vi "gxml_RcrsvParse.vi"(6 "File Item Contents":string, 7 "Empty XML Array?":bool, 8 "error in":errorcluster, 9 "Flat String In":string, 11 "Item TypeDesc":variant) -> (0 "error out":errorcluster, 1 "Flat String Out":string)   [LabVIEW 2011, in "Third Party VIs.lvlib" / "GXML.lvlib"]
doc: "This recursive VI is the core engine responsible for searching the XML string. The VI recursively dives into the type definition cluster and identifies individual elements by name. In parallel the VI also looks at the XML string for tags that have the same name and hierarchy. If a match is found the data is extracted from the XML file and appropriately inserted into a flattened data string."
uses:
  GXML.lvlib
  <vilib>/Utility/VariantDataType/VariantType.lvlib
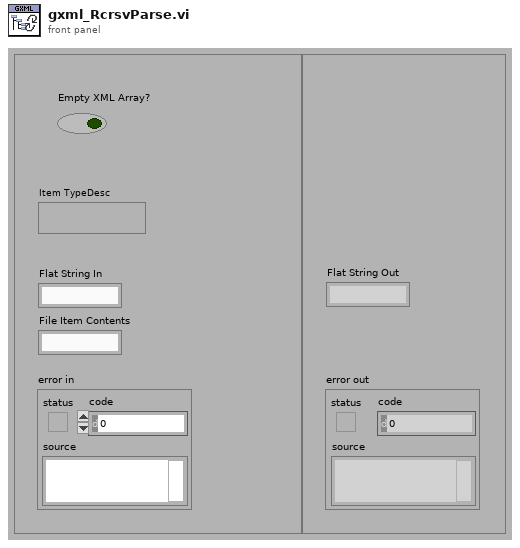
[diagram p1: front panel]
types:
  T1 = typedef "VariantType.lvlib/Type.ctl" = enum8{"Invalid Type", "Void", "I8", "I16", "I32", "I64", "U8", "U16", "U32", "U64", "Single Float", "Double Float", "Extended Float", "Single Complex", "Double Complex", "Extended Complex", "Enum U8", "Enum U16", "Enum U32", "Enum U64", "Single Float With Unit", "Double Float With Unit", "Extended Float With Unit", "Single Complex with Unit", "Double Complex with Unit", "Extended Complex with Unit", "Boolean", "String", "Path", "Picture", "Tag", "Array", "Cluster", "Variant", "LV Variant", "Waveform", "Timestamp", "Digital Waveform", "Digital Data", "ExpressData", "Refnum", "External Data", "VI", "Poly VI", "LabVIEW Class Instance", "Fixed Point"}
  T2 = cluster{"Item 'Name'":string, "Item Attributes":string, "Item Contents":string}
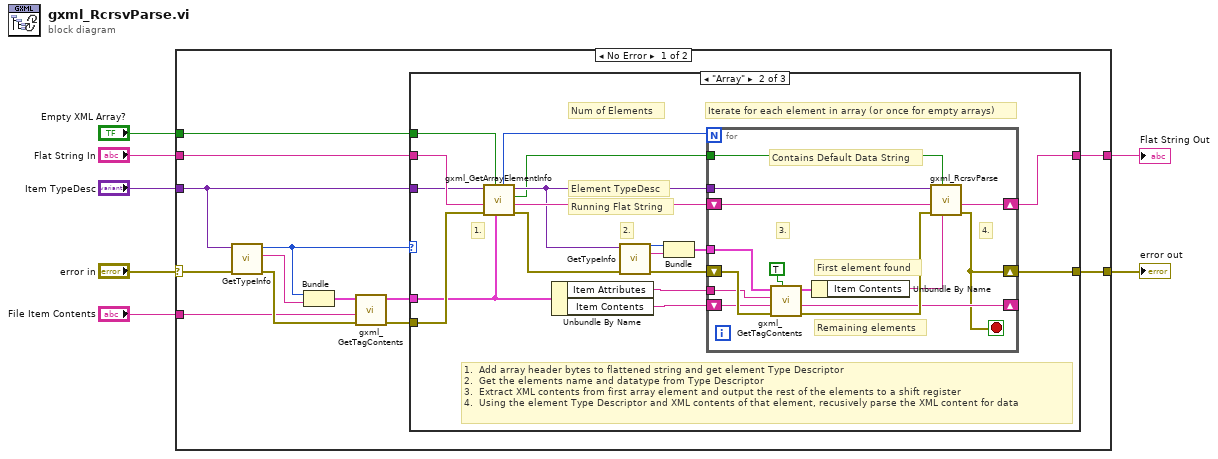
[diagram p0: block diagram]
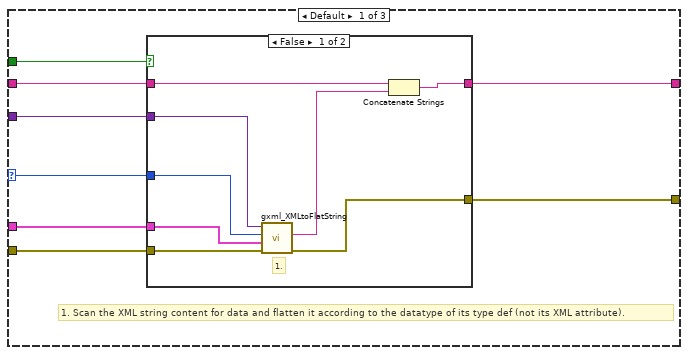
[diagram p2: hidden frame]
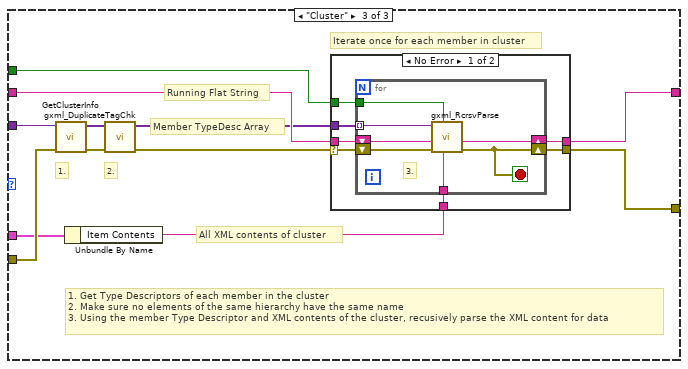
[diagram p4: hidden frame]
diagram:
  n1 = case shown="No Error" "error in" {
    selector: "error in" -> [w19 w100]
    tunnel: [w20 w100] -> w7
    tunnel: "File Item Contents" -> [w13 _]
    tunnel: "Item TypeDesc" -> [w18 _]
    tunnel: "Flat String In" -> [w9 w99]
    tunnel: [w17 w99] -> w3
    tunnel: "Empty XML Array?" -> [w8 _]
    frame No Error {
      n2 = call <vilib>:"GetTypeInfo.vi"("error in (no error)"=w19, "Variant"=w18) -> ("error out"=w16:errorcluster, "Name"=w10:string, "Type Enum"=w11:T1)  [unwired: 5 in, 2 out]
      n3 = Bundle("Type Enum"=w11, "Name"=w10) -> (w12:cluster{"Type Enum":T1, "Name":string})  [unwired: 1 in]
      n4 = call "gxml_GetTagContents.vi"("error in"=w16, "Item XML"=w13, "Item Name/Type"=w12) -> ("error out"=w15:errorcluster, "Item XML Data"=w14:T2)  [unwired: 6 in, 1 out]
      n5 = case shown="\"Array\"" w11 {
        selector: w11 -> [w26 _ _]
        tunnel: w18 -> [w27 w46 w82]
        tunnel: w15 -> [w28 w54 w81]
        tunnel: [w23 w55 w78] -> w20
        tunnel: w9 -> [w24 w49 w80]
        tunnel: [w22 w56 w79] -> w17
        tunnel: w14 -> [w25 w51 w77]
        tunnel: w8 -> [w21 w39 w75]
        frame Default {
          # "1. Scan the XML string content for data and flatten it according to the datatype of its type def (not its XML attribute)."
          n6 = case shown="False" w21 {
            tunnel: w28 -> [w36 w37]
            tunnel: w27 -> [w35 _]
            tunnel: w26 -> [w34 _]
            tunnel: w25 -> [w33 _]
            tunnel: w24 -> [w32 w38]
            tunnel: [w30 w37] -> w23
            tunnel: [w29 w38] -> w22
            frame False {
              # "1."
              n7 = call "gxml_XMLtoFlatString.vi"("error in"=w36, "Item XML Data"=w33, "Type Enum"=w34, "Item Type Desc"=w35) -> ("error out"=w30:errorcluster, "XML Data (Flat Str)"=w31:string)  [unwired: 6 in]
              n8 = Concatenate Strings(w32, w31) -> (w29:string)
            }
            frame True {
            }
          }
        }
        frame "Array" {
          # "Running Flat String"
          # "Element TypeDesc"
          # "Num of Elements"
          # "Iterate for each element in array (or once for empty arrays)"
          # "2."
          # "1."
          # "1.  Add array header bytes to flattened string and get element Type Descriptor\n2.  Get the elements name and datatype from Type Descriptor\n3.  Extract XML contents from first array element and output the rest of the elements to a shift register\n4.  Using the element Type Descriptor and XML contents of that element, recusively parse the XML content for data"
          n9 = call "gxml_GetArrayElementInfo.vi"("Item Data"=w51, "XML Array Empty?"=w39, "error in"=w54, "Flat String In"=w49, "Array TypeDesc"=w46) -> ("error out"=w48:errorcluster, "Flat String Out"=w50:string, "XML Array Empty?"=w40:bool, "Element TypeDesc"=w42:variant, "Element Count"=w41:i32)  [unwired: 2 in]
          n10 = Unbundle By Name(w51) -> ("Item Attributes"=w53:string, "Item Contents"=w52:string)
          n11 = call <vilib>:"GetTypeInfo.vi"("error in (no error)"=w48, "Variant"=w42) -> ("error out"=w47:errorcluster, "Name"=w44:string, "Type Enum"=w45:T1)  [unwired: 5 in, 2 out]
          n12 = Bundle("Type Enum"=w45, "Name"=w44) -> (w43:cluster{"Type Enum":T1, "Name":string})  [unwired: 1 in]
          n13 = for {
            N: w41 -> [_]
            tunnel: w42 -> [w59]
            shift-right: [w57] -> w56
            shift-left: w50 -> [w58]
            shift-right: [w67] -> _
            shift-left: w52 -> [w69]
            shift-right: [w66] -> w55
            shift-left: w47 -> [w70]
            tunnel: w53 -> [w65]
            tunnel: w43 -> [w61]
            tunnel: w40 -> [w60]
            stop <- w66 stop-if-true
            # "Contains Default Data String"
            # "Remaining elements"
            # "First element found"
            # "4."
            # "3."
            n14 = call "gxml_GetTagContents.vi"("Array Container?"=TRUE ("Include Tags?"), "error in"=w70, "Item XML"=w69, "Array Attributes"=w65, "Item Name/Type"=w61) -> ("error out"=w68:errorcluster, "XML After Closing Tag"=w67:string, "Item XML Data"=w63:T2)  [unwired: 4 in]
            n15 = Unbundle By Name(w63) -> ("Item Contents"=w62:string)
            n16 = call "gxml_RcrsvParse.vi"("File Item Contents"=w62, "Empty XML Array?"=w60, "error in"=w68, "Flat String In"=w58, "Item TypeDesc"=w59) -> ("error out"=w66:errorcluster, "Flat String Out"=w57:string)  [unwired: 5 in]
          }
        }
        frame "Cluster" {
          # "2."
          # "Member TypeDesc Array"
          # "Running Flat String"
          # "All XML contents of cluster"
          # "Iterate once for each member in cluster"
          # "1."
          # "1. Get Type Descriptors of each member in the cluster\n2. Make sure no elements of the same hierarchy have the same name \n3. Using the member Type Descriptor and XML contents of the cluster, recusively parse the XML content for data"
          n17 = call <vilib>:"GetClusterInfo.vi"("error in (no error)"=w81, "Variant"=w82) -> ("error out"=w74:errorcluster, "Cluster Elements"=w72:variant[])  [unwired: 8 in]
          n18 = Unbundle By Name(w77) -> ("Item Contents"=w76:string)
          n19 = call "gxml_DuplicateTagChk.vi"("error in"=w74, "Cluster Elements"=w72) -> ("error out"=w73:errorcluster, "Cluster Elements Out"=w71:variant[])  [unwired: 7 in]
          n20 = case shown="No Error" w73 {
            selector: w73 -> [w84 w98]
            tunnel: w80 -> [w89 w97]
            tunnel: w71 -> [w88 _]
            tunnel: w76 -> [w87 _]
            tunnel: [w86 w97] -> w79
            tunnel: [w85 w98] -> w78
            tunnel: w75 -> [w83 _]
            frame No Error {
              n21 = for {
                shift-right: [w90] -> w86
                shift-left: w89 -> [w91]
                tunnel: w88 -> [w92] mode=indexing
                tunnel: w87 -> [w94]
                shift-right: [w95] -> w85
                shift-left: w84 -> [w96]
                tunnel: w83 -> [w93]
                stop <- w95 stop-if-true
                # "3."
                n22 = call "gxml_RcrsvParse.vi"("File Item Contents"=w94, "Empty XML Array?"=w93, "error in"=w96, "Flat String In"=w91, "Item TypeDesc"=w92) -> ("error out"=w95:errorcluster, "Flat String Out"=w90:string)  [unwired: 5 in]
              }
            }
            frame Error {
            }
          }
        }
      }
    }
    frame Error {
    }
  }
  "error out" <- w7
  "Flat String Out" <- w3
